vi "FPGAoutput_fixed_8sample_x2.vi"() -> ()   [LabVIEW 2013]
uses:
  <vilib>/Platform/TimedLoop/XDataNode/timing_clust.ctl
  <vilib>/Platform/TimedLoop/XDataNode/nitl_modes.ctl
  <vilib>/Platform/TimedLoop/XDataNode/wakeup.ctl
  <vilib>/rvi/Emulation/niFpgaSctlEmulationGetInTimedLoop.vi
  <vilib>/rvi/Emulation/niFpgaEmulationReportErrorSimple.vi
  <vilib>/rvi/Emulation/niFpgaGetClockAttributes.vi
  <vilib>/rvi/eio/common/nirviEmuTemplateMethod_errors.vi
  <vilib>/rvi/Emulation/niFpgaCriticalErrorInLSC.vi
  <vilib>/Platform/TimedLoop/XDataNode/XDataNode.xnode
  <vilib>/eio/EIONode/EIONode.xnode
  <vilib>/Platform/TimedLoop/XDataNode/XDNodeRunTimeDep.lvlib
panel:
  in  "AO 0 N-7":i16
  in  "AO 0 N-6":i16
  in  "AO 0 N-5":i16
  in  "AO 0 N-4":i16
  in  "AO 0 N":i16
  in  "AO 0 N-1":i16
  in  "AO 0 N-2":i16
  in  "AO 0 N-3":i16
  out "IO Module\\Trigger Input":bool
  in  "User Command Commit":bool
  in  "User Command":u8
  out "User Command Idle":bool
  out "User Command Status":u8
  in  "User Data 0":u8
  in  "User Data 1":u8
  out "PLL Locked":bool
  out "User Error":bool
  out "Configured?":bool
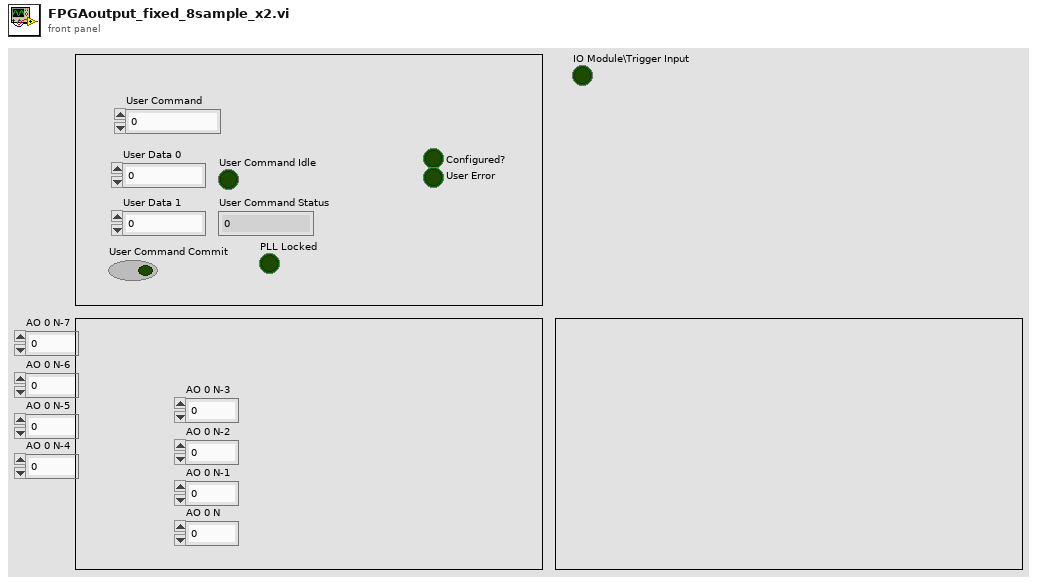
[diagram p1: front panel]
types:
  T1 = typedef "XDNodeRunTimeDep.lvlib/timing_clust.ctl" = cluster{"Expected End [f-1]":u64, "Actual End [f-1]":u64, "Finished Late? [f-1]":bool, "Expected End [i-1]":u64, "Actual End [i-1]":u64, "Finished Late? [i-1]":bool, "Expected Start [i]":u64, "Actual Start [i]":u64, "Expected Start [f]":u64, "Actual Start [f]":u64, "Source Name":string, "Structure Name":string, "Period":i64, "Deadline":i64, "Offset":i64, "Start":i64, "Priority":i32, "Timeout":i32, "Mode":T2, "Wakeup Reason":T3, "Error":errorcluster, "Source Type":string, "Secondary Source Type":string, "Global End Time":u64, "Global Start Time":u64, "Frame Duration":u64, "Iteration Duration":u64, "Assigned CPU":i32, "I/O Scan Engine Mode":u32}
  T2 = typedef "XDNodeRunTimeDep.lvlib/nitl_modes.ctl" = enum32{"No Change", "Process missed periods, maintain original phase", "Discard missed periods, maintain original phase", "Process missed periods, ignore original phase", "Discard missed periods, ignore original phase"}
  T3 = typedef "XDNodeRunTimeDep.lvlib/wakeup.ctl" = enum32{"Normal", "Aborted", "Asynchronous wakeup", "Timing source error", "Timed loop error", "Timeout"}
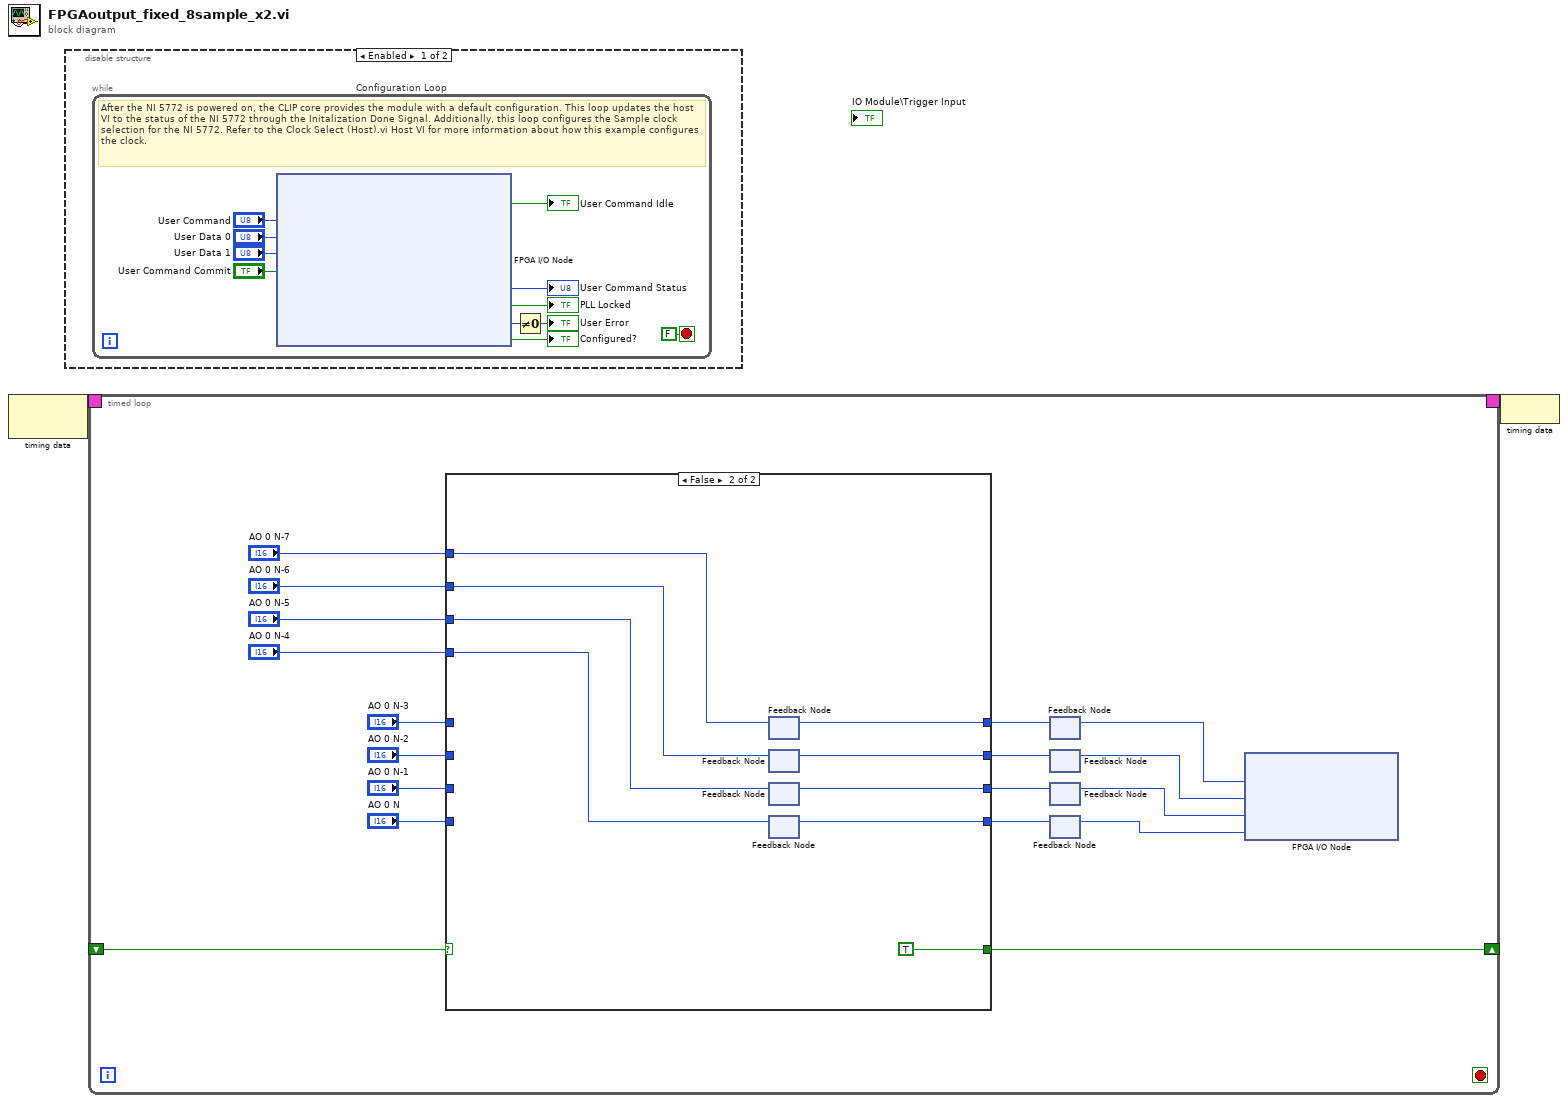
[diagram p0: block diagram]
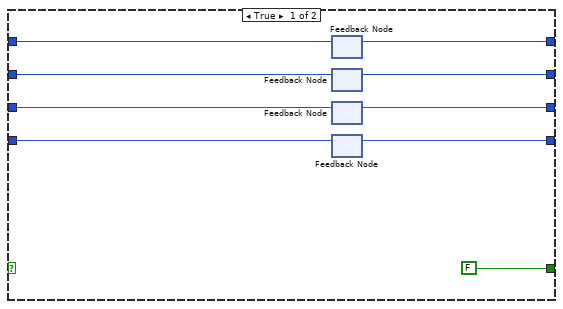
[diagram p2: hidden frame]
diagram:
  n1 = node-c288() -> (w2:T1)  [unwired: 1 in]
  n2 = disable-structure shown="Enabled" {
    frame Enabled {
      n3 = while "Configuration Loop" {
        stop <- FALSE stop-if-true
        # "After the NI 5772 is powered on, the CLIP core provides the module with a default configuration. This loop updates the host VI to the status of the NI 5772 through the Initalization Done Signal. Additionally, this loop configures the Sample clock selection for the NI 5772. Refer to the Clock Select (Host).vi Host VI for more information about how this example configures the clock."
        n4 = xnode "FPGA I/O Node"("IO Module\\User Command"="User Command", "IO Module\\User Data 0"="User Data 0", "IO Module\\User Data 1"="User Data 1", "IO Module\\User Command Commit"="User Command Commit") -> ("IO Module\\User Command Idle"=→"User Command Idle":bool, "IO Module\\User Command Status"=→"User Command Status":u8, "IO Module\\PLL Locked"=→"PLL Locked":bool, "IO Module\\User Error"=w8:u8, "IO Module\\Initialization Done"=→"Configured?":bool)  [unwired: 9 in, 9 out]
        n5 = Not Equal To 0?(x=w8) -> (x != 0?=→"User Error":bool)
      }
    }
    frame Disabled {
    }
  }
  n6 = timed-loop {
    timing: w2 -> [_]
    timing-out: [_] -> w1
    shift-right: [w27] -> _
    shift-left: _ -> [w26]
    stop <- _ stop-if-true
    n7 = case shown="False" w26 {
      tunnel: "AO 0 N-3" -> [w40 _]
      tunnel: "AO 0 N-2" -> [w39 _]
      tunnel: "AO 0 N-1" -> [w38 _]
      tunnel: "AO 0 N" -> [w37 _]
      tunnel: [FALSE TRUE] -> w27
      tunnel: "AO 0 N-7" -> [_ w44]
      tunnel: "AO 0 N-6" -> [_ w43]
      tunnel: "AO 0 N-5" -> [_ w42]
      tunnel: "AO 0 N-4" -> [_ w41]
      tunnel: [w35 w48] -> w17
      tunnel: [w34 w47] -> w16
      tunnel: [w33 w46] -> w15
      tunnel: [w32 w45] -> w14
      frame True {
        n8 = feedback #1() -> (w35:i16)  [unwired: 1 in]
        n9 = feedback-in #1(w40) -> ()
        n10 = feedback #2() -> (w34:i16)  [unwired: 1 in]
        n11 = feedback-in #2(w39) -> ()
        n12 = feedback #3() -> (w33:i16)  [unwired: 1 in]
        n13 = feedback-in #3(w38) -> ()
        n14 = feedback #4() -> (w32:i16)  [unwired: 1 in]
        n15 = feedback-in #4(w37) -> ()
      }
      frame False {
        n16 = feedback #5() -> (w48:i16)  [unwired: 1 in]
        n17 = feedback-in #5(w44) -> ()
        n18 = feedback #6() -> (w47:i16)  [unwired: 1 in]
        n19 = feedback-in #6(w43) -> ()
        n20 = feedback #7() -> (w46:i16)  [unwired: 1 in]
        n21 = feedback-in #7(w42) -> ()
        n22 = feedback #8() -> (w45:i16)  [unwired: 1 in]
        n23 = feedback-in #8(w41) -> ()
      }
    }
    n24 = feedback #9() -> (w18:i16)  [unwired: 1 in]
    n25 = feedback-in #9(w17) -> ()
    n26 = feedback #10() -> (w19:i16)  [unwired: 1 in]
    n27 = feedback-in #10(w16) -> ()
    n28 = feedback #11() -> (w20:i16)  [unwired: 1 in]
    n29 = feedback-in #11(w15) -> ()
    n30 = feedback #12() -> (w21:i16)  [unwired: 1 in]
    n31 = feedback-in #12(w14) -> ()
    n32 = xnode "FPGA I/O Node"("IO Module\\AO 0 N-3"=w18, "IO Module\\AO 0 N-2"=w19, "IO Module\\AO 0 N-1"=w20, "IO Module\\AO 0 N"=w21) -> ()  [unwired: 4 in, 4 out]
  }
  n33 = node-c288(w1) -> ()
